vi "Kalman_Filter_Gated_Filter.vi"(8 "error in (no error)":errorcluster, 11 "Kalman_Filter in":refnum<class "Kalman_Filter.lvclass">) -> (0 "error out":errorcluster, 3 "Kalman_Filter out":refnum<class "Kalman_Filter.lvclass">)   [LabVIEW 2021, in "Kalman_Filter.lvclass"]
uses:
  Kalman_Filter.lvclass
  Kalman_Filter.lvclass/Kalman_Filter.ctl
  <vilib>/Analysis/baseanly.llb/Real A x B.vi
  <vilib>/Analysis/Matrix/Numeric/Add/Add - RM,RM.vi
  <vilib>/Analysis/Matrix/Numeric/Add/Add (Elementwise) - RM,R.vi
  <vilib>/Analysis/Matrix/Numeric/Multiply/Multiply - RM,R.vi
  <vilib>/Analysis/Matrix/Numeric/Subtract/Subtract - RM,RM.vi
  <vilib>/Analysis/NI_AALBase.lvlib
  <vilib>/Analysis/Matrix/NI_Matrix.lvlib
panel:
  in  "New Measurement":dbl
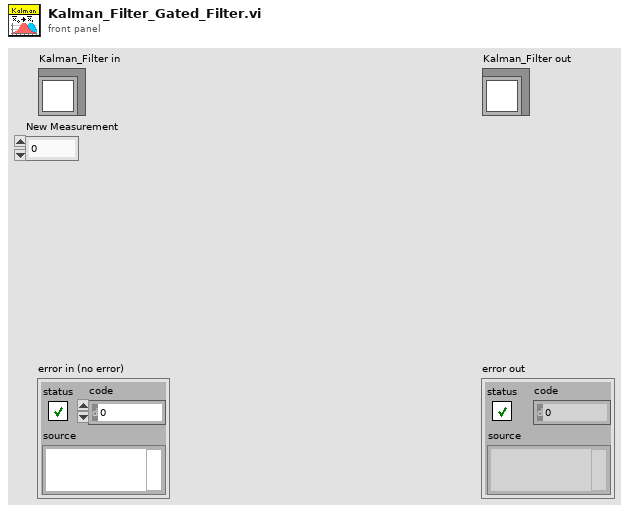
[diagram p1: front panel]
types:
  T1 = typedef "NI_Matrix.lvlib/RealMatrix.ctl" = dbl[][]
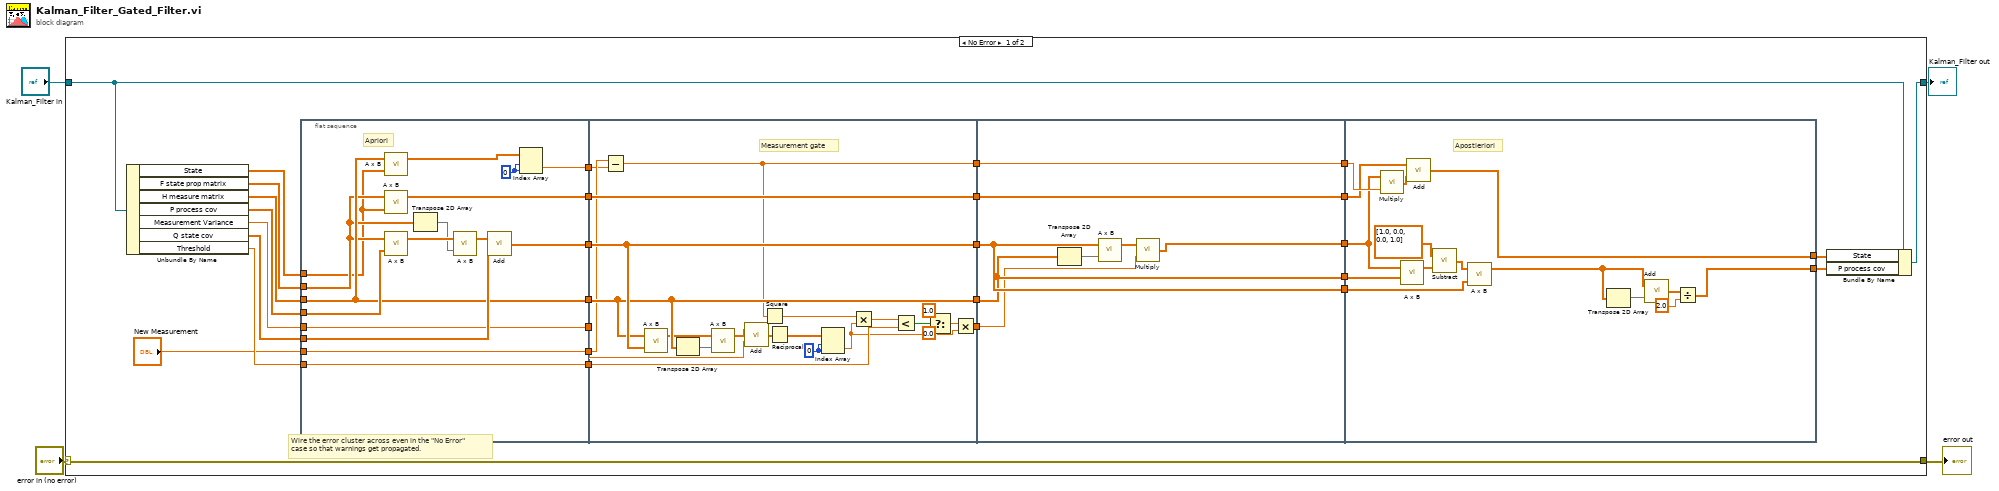
[diagram p0: block diagram]
diagram:
  n1 = case shown="No Error" "error in (no error)" {
    selector: "error in (no error)" -> [w34 w97]
    tunnel: [w34 w97] -> w3
    tunnel: "Kalman_Filter in" -> [w8 w96]
    tunnel: [w5 w96] -> w1
    frame No Error {
      # "Wire the error cluster across even in the \"No Error\"\ncase so that warnings get propagated."
      n2 = Unbundle By Name(w8) -> ("State"=w16:dbl[][], "F state prop matrix"=w15:dbl[][], "H measure matrix"=w14:dbl[][], "P process cov"=w13:dbl[][], "Measurement Variance"=w12:dbl, "Q state cov"=w11:dbl[][], "Threshold"=w10:dbl)
      n3 = flat-sequence {
        tunnel: w15 -> [w42]
        tunnel: w16 -> [w40]
        tunnel: w14 -> [w44]
        tunnel: [w35] -> w33
        tunnel: [w50] -> w32
        tunnel: "New Measurement" -> [w39]
        tunnel: w11 -> [w49]
        tunnel: w13 -> [w48]
        tunnel: [w45] -> w31
        tunnel: [w44] -> w30
        tunnel: w12 -> [w38]
        tunnel: [w38] -> w29
        tunnel: w10 -> [w43]
        tunnel: [w43] -> w28
        tunnel: [w39] -> w27
        tunnel: w33 -> [w51]
        tunnel: w32 -> [w72]
        tunnel: w31 -> [w70]
        tunnel: [w62] -> w26
        tunnel: w30 -> [w69]
        tunnel: w29 -> [w71]
        tunnel: [w72] -> w25
        tunnel: [w69] -> w24
        tunnel: [w70] -> w23
        tunnel: w28 -> [w68]
        tunnel: w27 -> [w52]
        tunnel: [w55] -> w22
        tunnel: w26 -> [w80]
        tunnel: [w80] -> w21
        tunnel: [w74] -> w20
        tunnel: w25 -> [w79]
        tunnel: [w79] -> w19
        tunnel: w24 -> [w77]
        tunnel: w23 -> [w78]
        tunnel: [w77] -> w18
        tunnel: [w78] -> w17
        tunnel: w22 -> [w75]
        tunnel: w21 -> [w95]
        tunnel: w20 -> [w91]
        tunnel: w19 -> [w93]
        tunnel: [w92] -> w7
        tunnel: w18 -> [w90]
        tunnel: w17 -> [w86]
        tunnel: [w81] -> w6
        frame #0 {
          w37 = 0 ("index (row)")
          # "Apriori"
          n4 = call-poly <vilib>:"A x B.vi"("B"=w40, "A"=w44) -> ("A x B"=w36:T1)  [unwired: 1 out]
          n5 = call-poly <vilib>:"A x B.vi"("B"=w40, "A"=w42) -> ("A x B"=w50:T1)  [unwired: 1 out]
          n6 = call-poly <vilib>:"A x B.vi"("B"=w48, "A"=w42) -> ("A x B"=w47:T1)  [unwired: 1 out]
          n7 = Transpose 2D Array(2D array=w42) -> (transposed array=w41:dbl[][])
          n8 = call-poly <vilib>:"A x B.vi"("B"=w41, "A"=w47) -> ("A x B"=w46:T1)  [unwired: 1 out]
          n9 = call-poly <vilib>:"Add.vi"("Real Matrix B"=w49, "Real Matrix A"=w46) -> ("A + B"=w45:T1)
          n10 = Index Array(array=w36, index (row)=w37, index (col)=w37) -> (element=w35:dbl)
        }
        frame #1 {
          w65 = 0 ("index (row)")
          # "Measurement gate"
          n11 = Subtract ("Subtract.vi")(x=w52, y=w51) -> (x-y=w62:dbl)
          n12 = call-poly <vilib>:"A x B.vi"("B"=w70, "A"=w69) -> ("A x B"=w67:T1)  [unwired: 1 out]
          n13 = Transpose 2D Array(2D array=w69) -> (transposed array=w66:dbl[][])
          n14 = call-poly <vilib>:"A x B.vi"("B"=w66, "A"=w67) -> ("A x B"=w63:T1)  [unwired: 1 out]
          n15 = call-poly <vilib>:"Add.vi"("Real Scalar c"=w71, "Real Matrix A"=w63) -> ("A + c"=w64:T1)
          n16 = Square(x=w62) -> (x^2=w61:dbl)
          n17 = Reciprocal(x=w64) -> (1/x=w59:T1)
          n18 = Index Array(array=w59, index (row)=w65, index (col)=w65) -> (element=w53:dbl)
          n19 = Multiply ("Multiply.vi")(x=w61, y=w53) -> (x*y=w60:dbl)
          n20 = Less?(x=w60, y=w68) -> (x < y?=w58:bool)
          n21 = Select(t=1.0, s=w58, f=0.0) -> (s? t:f=w54:dbl)
          n22 = Multiply(x=w54, y=w53) -> (x*y=w55:dbl)
        }
        frame #2 {
          n23 = Transpose 2D Array(2D array=w77) -> (transposed array=w76:dbl[][])
          n24 = call-poly <vilib>:"A x B.vi"("B"=w76, "A"=w78) -> ("A x B"=w73:T1)  [unwired: 1 out]
          n25 = call-poly <vilib>:"Multiply.vi"("Real Scalar c"=w75, "Real Matrix A"=w73) -> ("A * c"=w74:T1)
        }
        frame #3 {
          # "Apostieriori"
          n26 = call-poly <vilib>:"Multiply.vi"("Real Scalar c"=w95, "Real Matrix A"=w91) -> ("A * c"=w94:T1)
          n27 = call-poly <vilib>:"A x B.vi"("B"=w90, "A"=w91) -> ("A x B"=w88:T1)  [unwired: 1 out]
          n28 = call-poly <vilib>:"Add.vi"("Real Matrix B"=w94, "Real Matrix A"=w93) -> ("A + B"=w92:T1)
          n29 = call-poly <vilib>:"Subtract.vi"("Real Matrix B"=w88, "Real Matrix A"=dbl[][] [[1.0, 0.0], [0.0, 1.0]]) -> ("A - B"=w87:T1)
          n30 = call-poly <vilib>:"A x B.vi"("B"=w86, "A"=w87) -> ("A x B"=w82:T1)  [unwired: 1 out]
          n31 = Transpose 2D Array(2D array=w82) -> (transposed array=w85:T1)
          n32 = call-poly <vilib>:"Add.vi"("Real Matrix B"=w85, "Real Matrix A"=w82) -> ("A + B"=w84:T1)
          n33 = Divide(x=w84, y=2.0) -> (x/y=w81:T1)
        }
      }
      n34 = Bundle By Name(cluster=w8, "State"=w7, "P process cov"=w6) -> (w5:refnum<class "Kalman_Filter.lvclass">)
    }
    frame Error {
    }
  }
  "error out" <- w3
  "Kalman_Filter out" <- w1
